vi "generate_16bit_sample.vi"(4 "Value":u16) -> (0 "latch":digitalwaveform(graph), 1 "clock":digitalwaveform(graph), 2 "data":digitalwaveform(graph))   [LabVIEW 2013]
uses:
  <vilib>/Waveform/DWDTOps.llb/Digital Pattern Generator (Single Value).vi
  <vilib>/Waveform/DWDTOps.llb/DWDT Append Digital Samples.vi
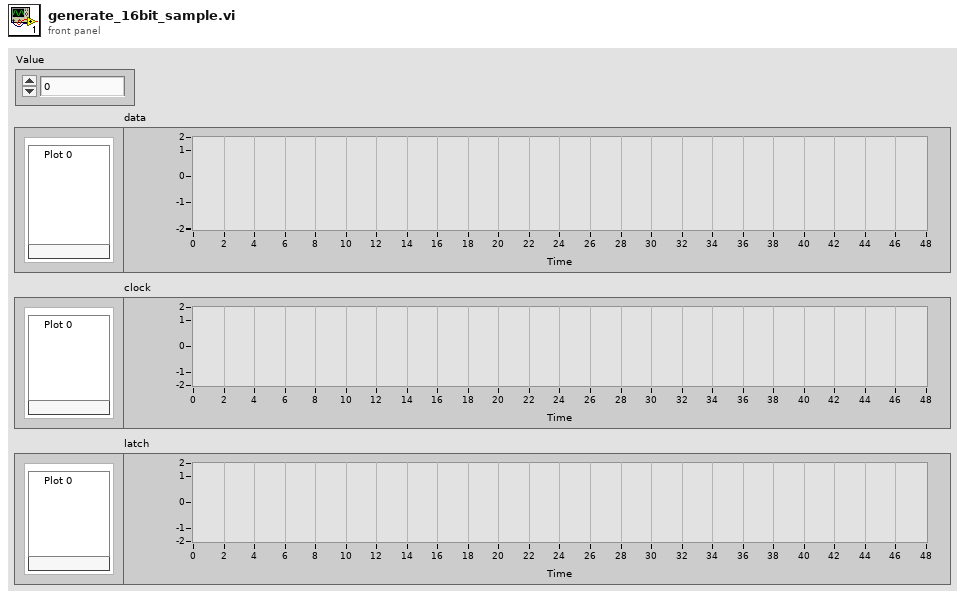
[diagram p1: front panel]
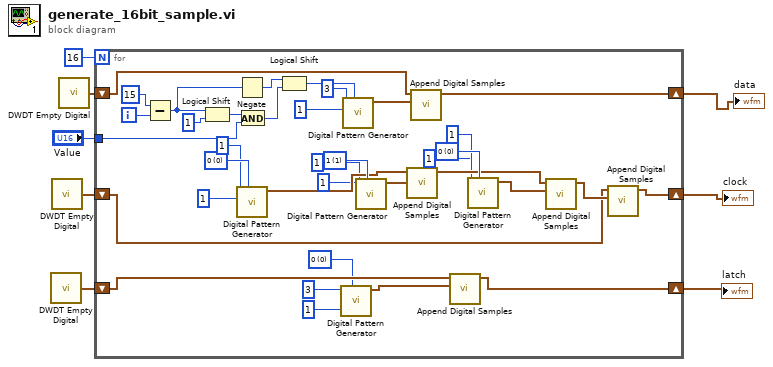
[diagram p0: block diagram]
diagram:
  n1 = call <vilib>:"DWDT Empty Digital.vi"() -> ("digital waveform out"=w4:digitalwaveform)  [unwired: 5 in]
  n2 = call <vilib>:"DWDT Empty Digital.vi"() -> ("digital waveform out"=w5:digitalwaveform)  [unwired: 5 in]
  n3 = call <vilib>:"DWDT Empty Digital.vi"() -> ("digital waveform out"=w6:digitalwaveform)  [unwired: 5 in]
  n4 = for {
    N: 16 -> [_]
    tunnel: "Value" -> [w40]
    shift-right: [w33] -> w3
    shift-left: w6 -> [w34]
    shift-right: [w21] -> w2
    shift-left: w5 -> [w15]
    shift-right: [w28] -> w1
    shift-left: w4 -> [w29]
    i -> [w43]
    w22 = u8 0 items=["0", "1", "Z", "L", "H", "X", "T", "V"] ("value")
    w23 = u8 1 items=["0", "1", "Z", "L", "H", "X", "T", "V"] ("value")
    w24 = u8 0 items=["0", "1", "Z", "L", "H", "X", "T", "V"] ("value")
    w27 = u8 0 items=["0", "1", "Z", "L", "H", "X", "T", "V"] ("value")
    n5 = Subtract(x=u16 15, y=w43) -> (x-y=w39:i32)
    n6 = Logical Shift(y=w39, x=u32 1) -> (x << y=w41:u32)
    n7 = Negate(x=w39) -> (-x=w38:i32)
    n8 = call-poly <vilib>:"Digital Pattern Generator.vi"("value"=w24, "number of signals"=u32 1, "number of samples"=u32 1) -> ("digital waveform"=w20:digitalwaveform)  [unwired: 7 in, 1 out]
    n9 = And(x=w41, y=w40) -> (x .and. y?=w37:u32)
    n10 = Logical Shift(y=w38, x=w37) -> (x << y=w36:u32)
    n11 = call-poly <vilib>:"Digital Pattern Generator.vi"("value"=w27, "number of signals"=u32 1, "number of samples"=u32 3) -> ("digital waveform"=w30:digitalwaveform)  [unwired: 7 in, 1 out]
    n12 = call-poly <vilib>:"Digital Pattern Generator.vi"("value"=w36, "number of signals"=u32 1, "number of samples"=u32 3) -> ("digital waveform"=w35:digitalwaveform)  [unwired: 7 in, 1 out]
    n13 = call-poly <vilib>:"Digital Pattern Generator.vi"("value"=w23, "number of signals"=u32 1, "number of samples"=u32 1) -> ("digital waveform"=w19:digitalwaveform)  [unwired: 7 in, 1 out]
    n14 = call-poly <vilib>:"Append Digital Samples.vi"("digital waveform B"=w19, "digital waveform A"=w20) -> ("digital waveform out"=w18:digitalwaveform)  [unwired: 8 in, 1 out]
    n15 = call-poly <vilib>:"Append Digital Samples.vi"("digital waveform B"=w35, "digital waveform A"=w34) -> ("digital waveform out"=w33:digitalwaveform)  [unwired: 8 in, 1 out]
    n16 = call-poly <vilib>:"Append Digital Samples.vi"("digital waveform B"=w30, "digital waveform A"=w29) -> ("digital waveform out"=w28:digitalwaveform)  [unwired: 8 in, 1 out]
    n17 = call-poly <vilib>:"Digital Pattern Generator.vi"("value"=w22, "number of signals"=u32 1, "number of samples"=u32 1) -> ("digital waveform"=w17:digitalwaveform)  [unwired: 7 in, 1 out]
    n18 = call-poly <vilib>:"Append Digital Samples.vi"("digital waveform B"=w17, "digital waveform A"=w18) -> ("digital waveform out"=w16:digitalwaveform)  [unwired: 8 in, 1 out]
    n19 = call-poly <vilib>:"Append Digital Samples.vi"("digital waveform B"=w16, "digital waveform A"=w15) -> ("digital waveform out"=w21:digitalwaveform)  [unwired: 8 in, 1 out]
  }
  "data" <- w3
  "clock" <- w2
  "latch" <- w1
